vi "Actor Core.vi"(8 "error in":errorcluster, 11 "Analyzing Dialog View in":refnum<class "Analyzing Dialog View.lvclass">) -> (0 "error out":errorcluster, 3 "Actor out":refnum<class "Actor.lvclass">)   [LabVIEW 2013, in "Analyzing Dialog View.lvlib" / "Analyzing Dialog View.lvclass"]
doc: "(<B>Filename</B>: Actor Framework.lvlib:Actor.lvclass:Actor Core.vi)\n\nReceives messages to the actor, reacts to them, and initiates any error handling that may shut the actor down.\n\nDescendant classes may override this VI to append parallel tasks for the actor to complete while it handles messages. Overrides use the Call Parent Method node."
uses:
  Analyzing Dialog View.lvclass
  <vilib>/ActorFramework/Actor/Actor.lvclass
  <vilib>/ActorFramework/Actor/Actor.lvclass/Actor.ctl
  <vilib>/ActorFrameworkMVC/View Actor/View Actor.lvclass
panel:
  out "Message":string="正在分析…"
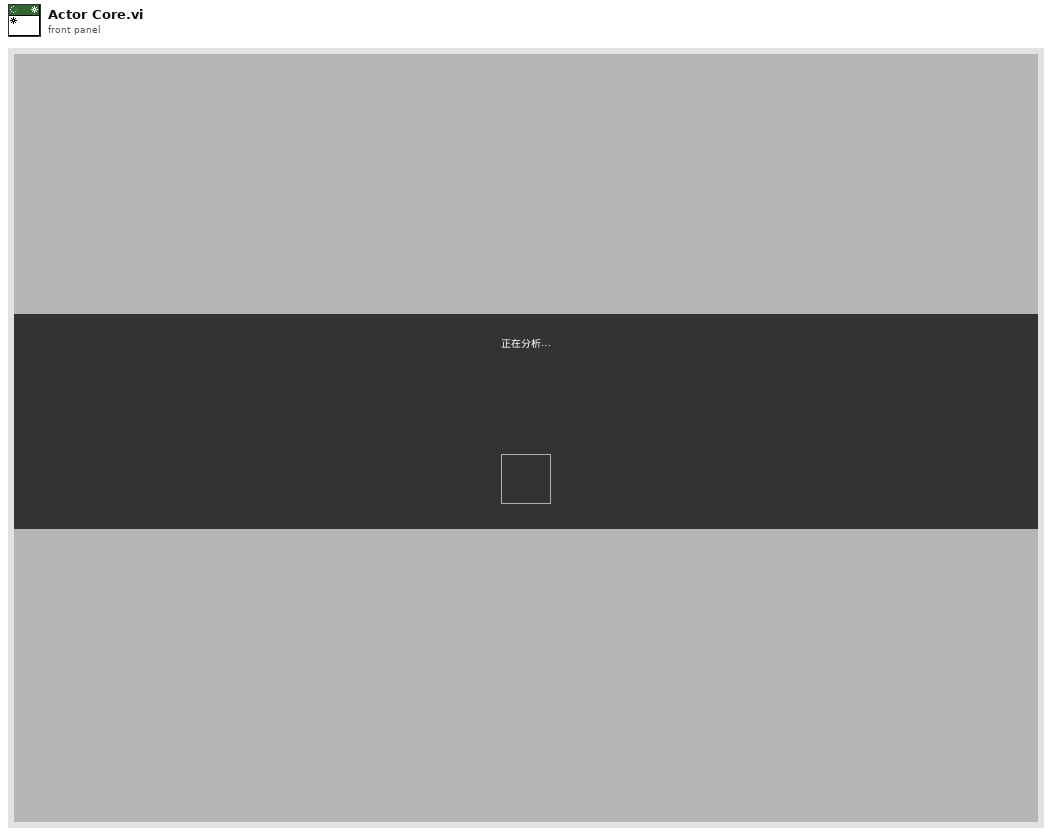
[diagram p1: front panel]
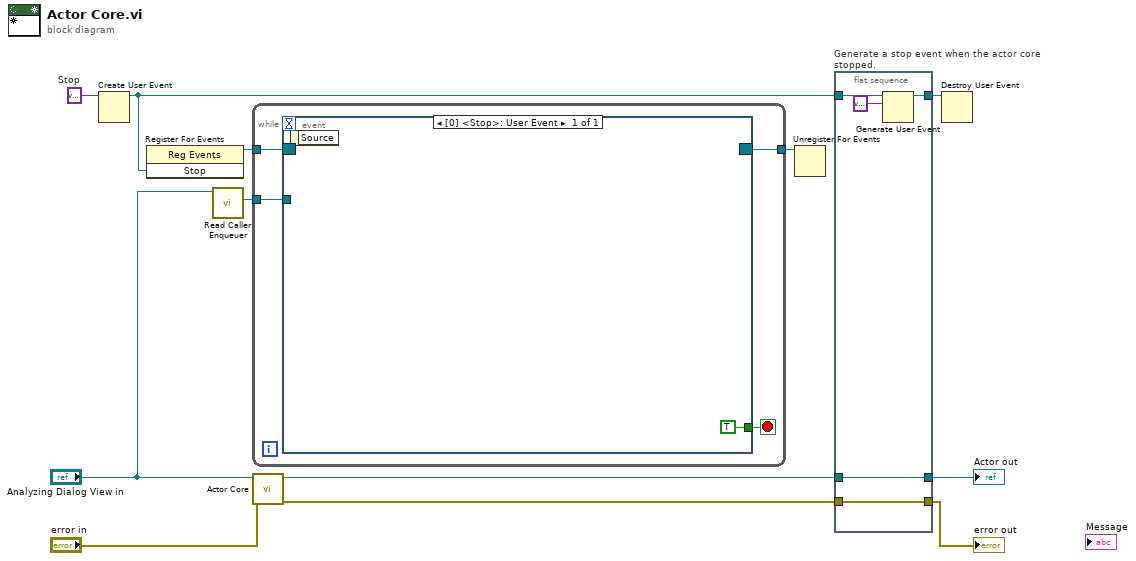
[diagram p0: block diagram]
diagram:
  w12 = variant  # Stop
  n1 = Create User Event(user event datatype=w12) -> (user event=w4:refnum<user-event>)  [unwired: 1 in, 1 out]
  n2 = register-events(w4) -> (reference out=w5:refnum<event-registration>)  [unwired: 2 in, 1 out]
  n3 = call <vilib>:"Read Caller Enqueuer.vi"("Actor"="Analyzing Dialog View in") -> ("Caller Enqueuer"=w2:refnum<class "Message Enqueuer.lvclass">)  [unwired: 10 in]
  n4 = while {
    tunnel: [w16] -> w3
    tunnel: w5 -> [w14]
    tunnel: w2 -> [w13]
    stop <- w15 stop-if-true
    n5 = event shown="[0] <Stop>: User Event" {
      selector: w14 -> [_]
      dyn-events: [_] -> w16
      timeout: _ -> [_]
      tunnel: [TRUE] -> w15
      tunnel: w13 -> [_]
      event User Event {
        n6 = event-data() -> ()  [unwired: 1 in, 1 out]
      }
    }
  }
  n7 = call-parent "Actor Core.vi"("error in"="error in", "View Actor in"="Analyzing Dialog View in") -> ("error out"=w8:errorcluster, "Actor out"=w9:refnum<class "Actor.lvclass">)  [unwired: 8 in]
  n8 = Unregister For Events(event registration refnum=w3) -> ()  [unwired: 1 in, 1 out]
  n9 = flat-sequence "Generate a stop event when the actor core stopped." {
    tunnel: w4 -> [w22]
    tunnel: [w20] -> w11
    tunnel: w9 -> [w19]
    tunnel: w8 -> [w18]
    tunnel: [w19] -> w7
    tunnel: [w18] -> w6
    frame #0 {
      n10 = Generate User Event(user event=w22, event data cluster=variant ("event data")) -> (user event out=w20:refnum<user-event>)  [unwired: 2 in, 1 out]
    }
  }
  n11 = Destroy User Event(user event=w11) -> ()  [unwired: 1 in, 1 out]
  "error out" <- w6
  "Actor out" <- w7
